vi "CmdConsole.Check Running State.vi"(8 "error in (no error)":errorcluster, 11 "CmdConsole in":refnum<class "CmdConsole.lvclass">) -> (0 "error out":errorcluster, 2 "Running":bool, 3 "CmdConsole out":refnum<class "CmdConsole.lvclass">)   [LabVIEW 2018, in "CmdConsole.lvclass"]
uses:
  CmdConsole.lvclass
  CmdConsole.lvclass/CmdConsole.ctl
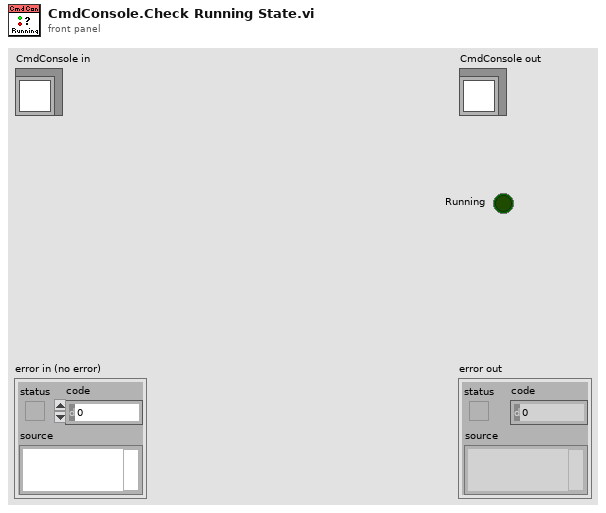
[diagram p1: front panel]
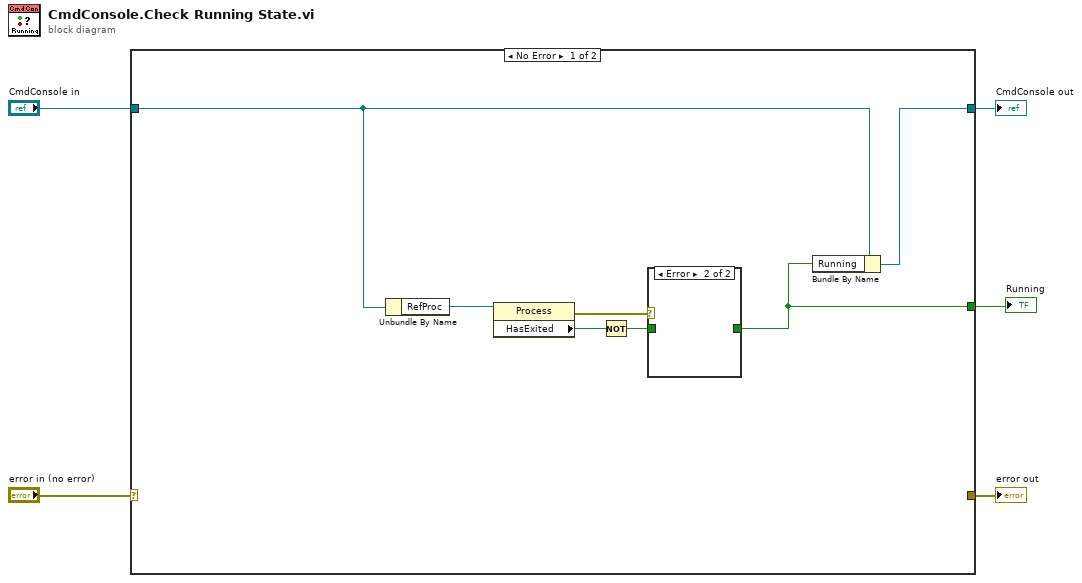
[diagram p0: block diagram]
diagram:
  n1 = case shown="No Error" "error in (no error)" {
    selector: "error in (no error)" -> [_ w15]
    tunnel: [_ w15] -> w4
    tunnel: [w9 w14] -> w2
    tunnel: "CmdConsole in" -> [w10 w14]
    tunnel: [w6 _] -> w1
    frame No Error {
      n2 = Unbundle By Name(w10) -> ("RefProc"=w12:refnum<k24>)
      n3 = property class="Process"(reference=w12) -> (error out=w8:errorcluster, "HasExited"=w11:bool)  [unwired: 1 in, 1 out]
      n4 = Not(x=w11) -> (.not. x?=w7:bool)
      n5 = case shown="Error" w8 {
        tunnel: w7 -> [w13 _]
        tunnel: [w13 _] -> w6
        frame No Error {
        }
        frame Error {
        }
      }
      n6 = Bundle By Name(cluster=w10, "Running"=w6) -> (w9:refnum<class "CmdConsole.lvclass">)
    }
    frame Error {
    }
  }
  "error out" <- w4
  "CmdConsole out" <- w2
  "Running" <- w1
